vi "Sans titre 1.vi"() -> ()   [LabVIEW 2024]
panel:
  out "chaîne concaténée":string
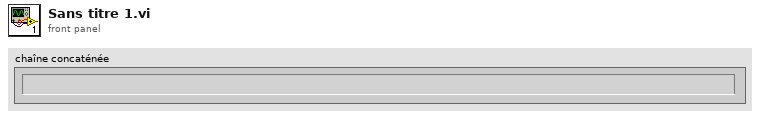
[diagram p1: front panel]
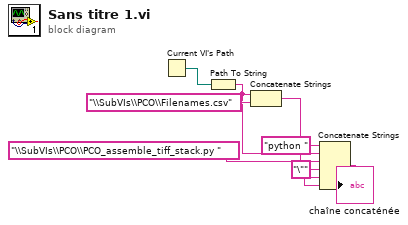
[diagram p0: block diagram]
diagram:
  w2 = "\"" ("chaîne")
  n1 = Current VI's Path() -> (path=w8:path)
  n2 = Path To String(path=w8) -> (string=w5:string)
  n3 = Concatenate Strings(w5, "\\SubVIs\\PCO\\Filenames.csv" ("chaîne")) -> (w3:string)
  n4 = Concatenate Strings("python " ("chaîne"), w5, "\\SubVIs\\PCO\\PCO_assemble_tiff_stack.py " ("chaîne"), w2, w3, w2) -> (→"chaîne concaténée":string)
